vi "Error Reporting Test.vi"(8 "error in (no error)":errorcluster, 11 "Async Actor Example in":refnum<class "Async Methods Actor Example.lvclass">) -> (0 "error out":errorcluster, 3 "Async Actor Example out":refnum<class "Async Methods Actor Example.lvclass">)   [LabVIEW 2023, in "Async Methods Actor Example.lvlib" / "Async Methods Actor Example.lvclass"]
uses:
  Async Methods Actor Example.lvclass
  Async Methods Actor Example.lvclass/Async Methods Actor Example.ctl
  <vilib>/Utility/error.llb/Error Cluster From Error Code.vi
  <vilib>/ErrorRing/Error Ring.xnode
panel:
  in  "Exit WIth Error":bool
  in  "Stop":bool
  out "String":string
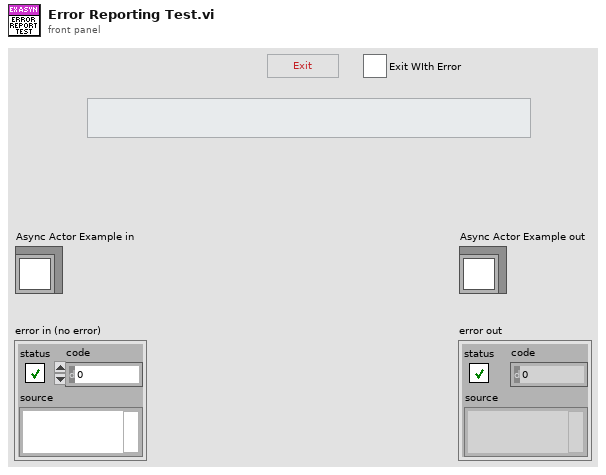
[diagram p1: front panel]
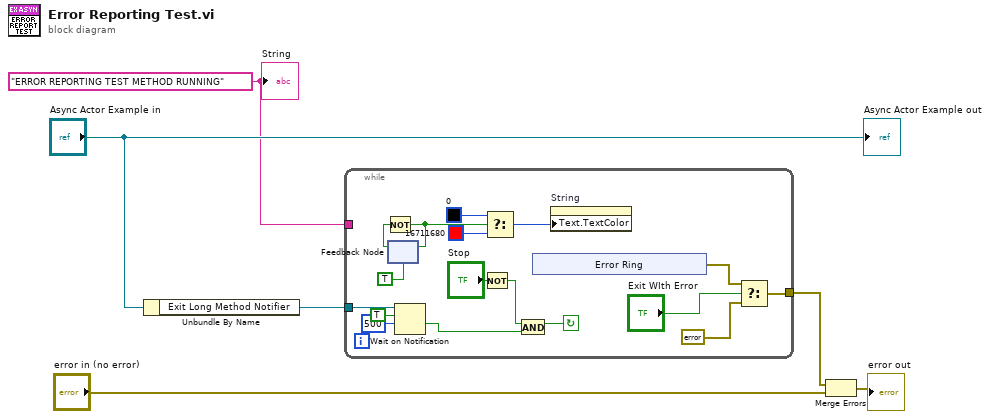
[diagram p0: block diagram]
diagram:
  w3 = "ERROR REPORTING TEST METHOD RUNNING" ("String")
  n1 = Unbundle By Name("Async Actor Example in") -> ("Exit Long Method Notifier"=w4:refnum<notifier>)
  n2 = while {
    tunnel: w4 -> [w17]
    tunnel: w3 -> [_]
    tunnel: [w7] -> w1
    stop <- w15 continue-if-true
    n3 = feedback #1(TRUE) -> (w22:bool)
    n4 = Not(x=w22) -> (.not. x?=w21:bool)
    n5 = feedback-in #1(w21) -> ()
    n6 = Wait on Notification(notifier=w17, ignore previous (F)=TRUE, timeout in ms (-1)=500) -> (timed out?=w14:bool)  [unwired: 1 in, 3 out]
    n7 = Not(x="Stop") -> (.not. x?=w12:bool)
    n8 = Select(t=u32 0 ("Text.Text Colors:Text Color"), s=w21, f=u32 16711680 ("Text.Text Colors:Text Color")) -> (s? t:f=w18:u32)
    n9 = And(x=w12, y=w14) -> (x .and. y?=w15:bool)
    n10 = xnode "Error Ring"() -> ("error out"=w10:errorcluster)
    n11 = property on="String" class="Str"("Text.TextColor"=w18) -> ()  [unwired: 2 in, 2 out]
    n12 = Select(t=w10, s="Exit WIth Error", f=errorcluster {"status"=FALSE, "code"=0, "source"=""}) -> (s? t:f=w7:errorcluster)
  }
  n13 = Merge Errors(w1, "error in (no error)") -> (→"error out":errorcluster)
  "Async Actor Example out" <- "Async Actor Example in"
  "String" <- w3
